vi "Create New Branch.vi"(8 "error in":errorcluster, 10 "Branch Data":variant, 11 "Name":string) -> (0 "error out":errorcluster, 3 "Tree out":refnum<class "Tree.lvclass">)   [LabVIEW 2019, in "Tree.lvclass"]
uses:
  Tree.lvclass
  Tree.lvclass/Tree.ctl
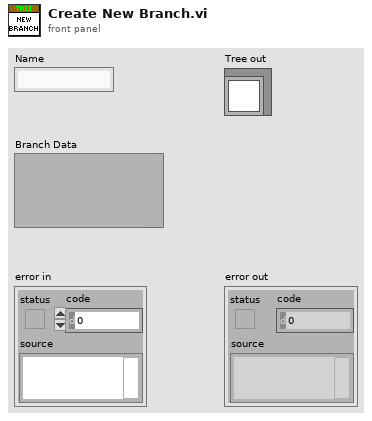
[diagram p1: front panel]
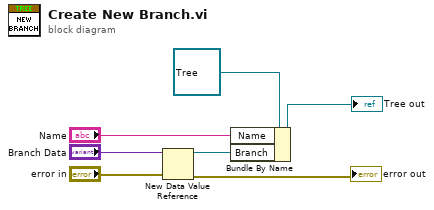
[diagram p0: block diagram]
diagram:
  n1 = New Data Value Reference(data value="Branch Data", error in="error in") -> (data value reference=w5:refnum<data-value>, error out=→"error out":errorcluster)
  n2 = Bundle By Name(cluster=refnum<class "Tree.lvclass"> refnum ("Tree out"), "Name"="Name", "Branch"=w5) -> (→"Tree out":refnum<class "Tree.lvclass">)
